vi "sub_font_customize.vi"(0 "REF IN":refnum<vi>, 1 "NOTE":string, 2 "FONT STYLE":T1, 3 "FONT COLOR":cluster{"COLOR":u32, "PHRASE":string[]}[](array[cluster]), 5 "ERROR IN":errorcluster, 8 "HEADER":string, 10 "HEADER EN?":bool) -> (14 "REF OUT":refnum<vi>, 19 "ERROR OUT":errorcluster)   [LabVIEW 2018]
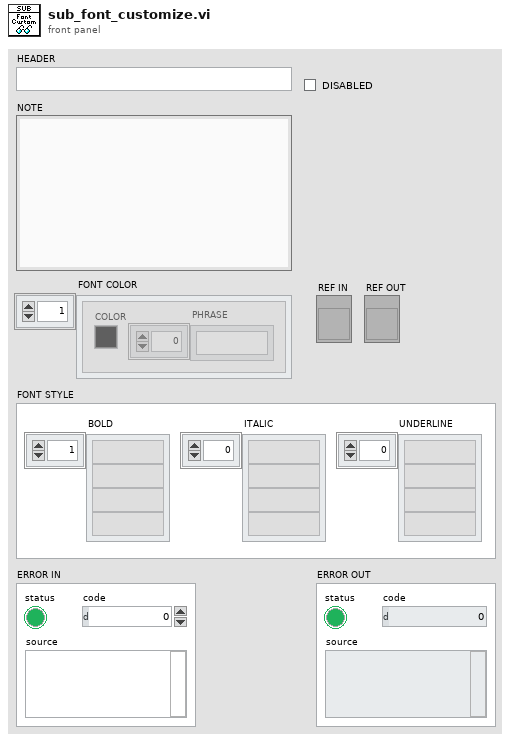
[diagram p1: front panel]
types:
  T1 = cluster{"BOLD":string[], "ITALIC":string[], "UNDERLINE":string[]}
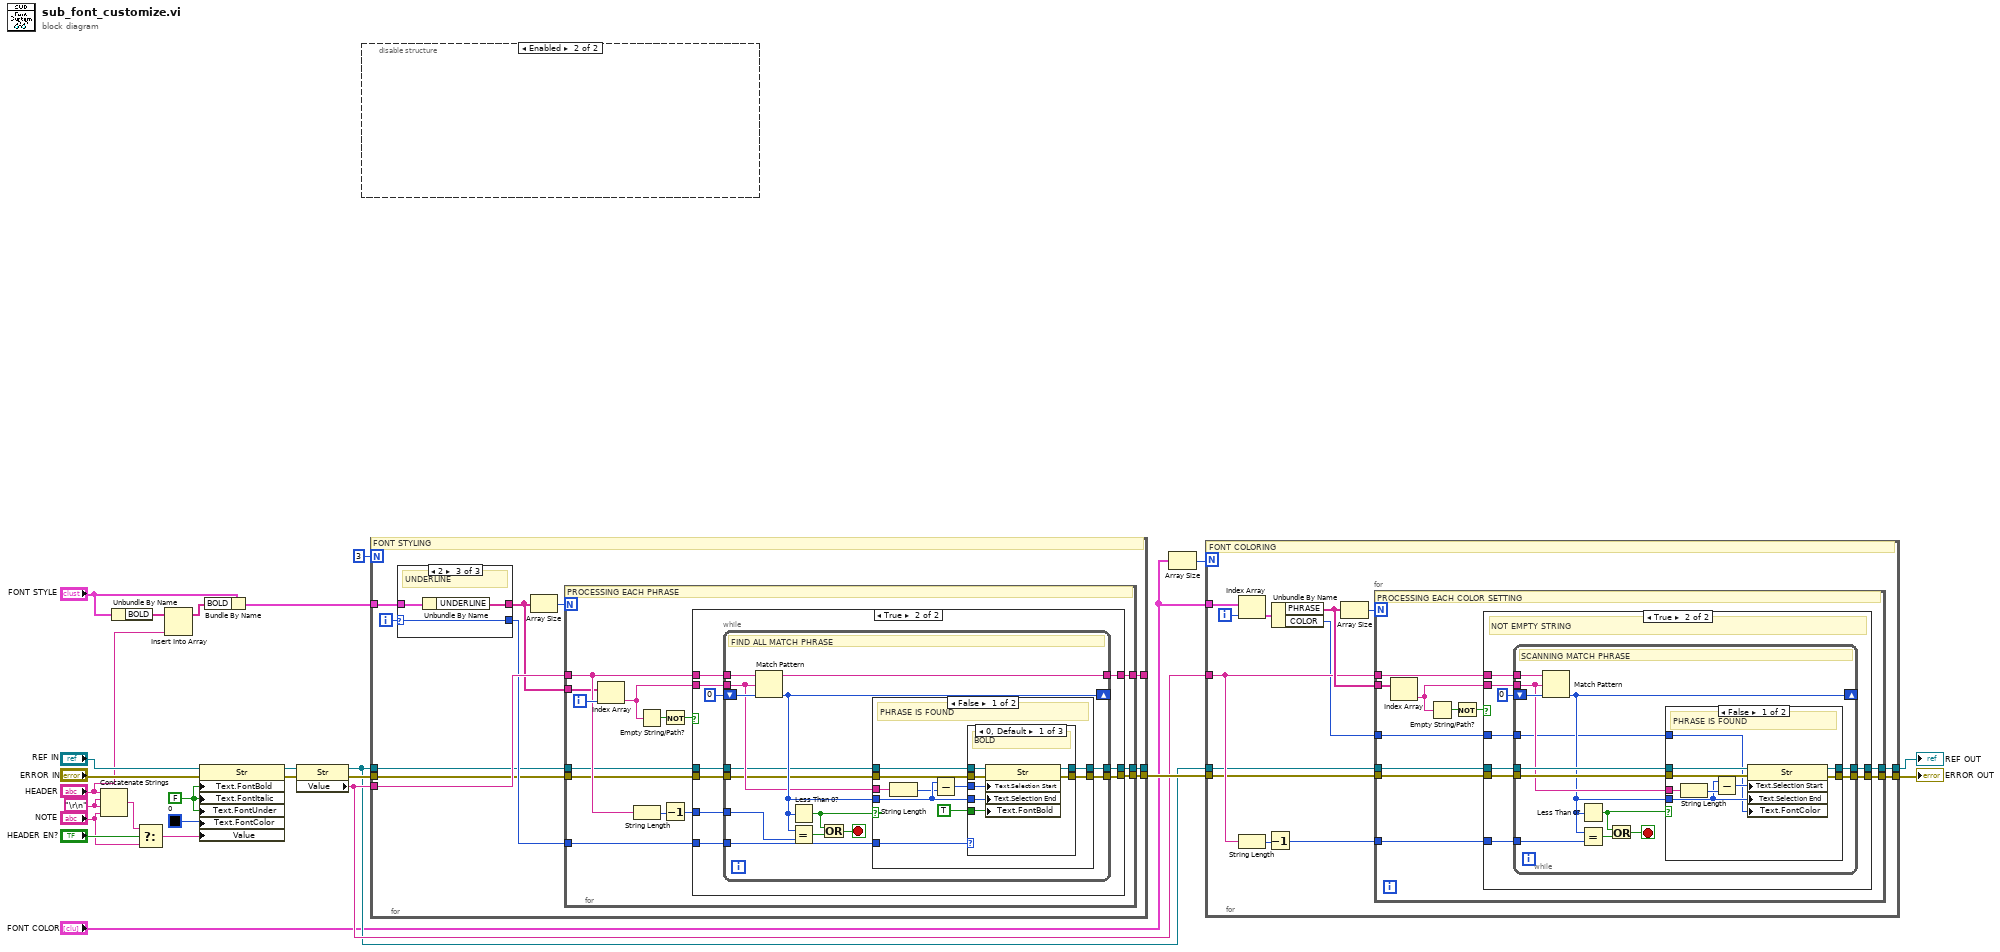
[diagram p0: block diagram]
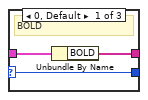
[diagram p4: hidden frame]
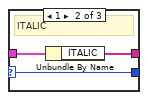
[diagram p5: hidden frame]
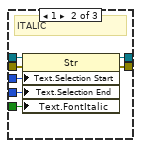
[diagram p7: hidden frame]
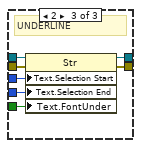
[diagram p8: hidden frame]
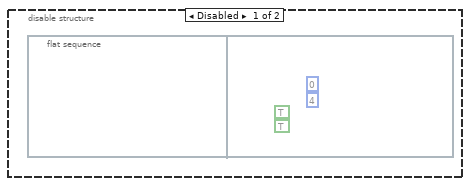
[diagram p10: hidden frame]
diagram:
  w11 = "\r\n"
  w25 = FALSE ("Text.Font:Bold")
  n1 = Concatenate Strings("HEADER", w11, w11, "NOTE") -> (w10:string)
  n2 = Unbundle By Name("FONT STYLE") -> ("BOLD"=w5:string[])
  n3 = Select(t=w10, s="HEADER EN?", f="NOTE") -> (s? t:f=w8:string)
  n4 = Insert Into Array(array=w5, new element="HEADER") -> (w2:string[])  [unwired: 1 in]
  n5 = property on="Property Node" class="Str"(reference="REF IN", error in="ERROR IN", "Text.FontBold"=w25, "Text.FontItalic"=w25, "Text.FontUnder"=w25, "Text.FontColor"=u32 0, "Value"=w8) -> (reference out=w20:refnum<vi>, error out=w23:errorcluster)
  n6 = Bundle By Name(cluster="FONT STYLE", "BOLD"=w2) -> (w1:T1)
  n7 = property on="Property Node" class="Str"(reference=w20, error in=w23) -> (reference out=w15:refnum<vi>, error out=w21:errorcluster, "Value"=w16:string)
  n8 = disable-structure shown="Enabled" {
    frame Disabled {
      n9 = flat-sequence {
        frame #0 {
        }
        frame #1 {
          w26 = TRUE ("Text.Font:Underline")
          w27 = TRUE ("Text.Font:Bold")
          w28 = u32 4 ("Text.Selection:End")
          w29 = u32 0 ("Text.Selection:Start")
        }
      }
    }
    frame Enabled {
    }
  }
  n10 = for {
    N: 3 -> [_]
    tunnel: w16 -> [w40]
    tunnel: w1 -> [w39]
    tunnel: w21 -> [w34]
    tunnel: w15 -> [w33]
    tunnel: [w32] -> _
    tunnel: [w31] -> w18
    tunnel: [w30] -> _
    i -> [w38]
    # "FONT STYLING"
    n11 = case shown="2" w38 {
      selector: w38 -> [w41 w44 w47]
      tunnel: w39 -> [w43 w46 w49]
      tunnel: [w42 w45 w48] -> w36
      tunnel: [w41 w44 w47] -> w37
      frame 0, Default {
        # "BOLD"
        n12 = Unbundle By Name(w43) -> ("BOLD"=w42:string[])
      }
      frame 1 {
        # "ITALIC"
        n13 = Unbundle By Name(w46) -> ("ITALIC"=w45:string[])
      }
      frame 2 {
        # "UNDERLINE"
        n14 = Unbundle By Name(w49) -> ("UNDERLINE"=w48:string[])
      }
    }
    n15 = Array Size(array=w36) -> (size(s)=w35:i32)
    n16 = for {
      N: w35 -> [_]
      tunnel: w40 -> [w60]
      tunnel: w34 -> [w59]
      tunnel: [w58] -> w31
      tunnel: [w57] -> w30
      tunnel: w37 -> [w56]
      tunnel: w36 -> [w55]
      tunnel: w33 -> [w51]
      tunnel: [w50] -> w32
      i -> [w63]
      # "PROCESSING EACH PHRASE"
      n17 = Index Array(array=w55, index=w63) -> (element=w54:string)
      n18 = String Length(string=w60) -> (length=w62:i32)
      n19 = Empty String/Path?(string/path=w54) -> (empty?=w52:bool)
      n20 = Not(x=w52) -> (.not. x?=w53:bool)
      n21 = Decrement(x=w62) -> (x-1=w61:i32)
      n22 = case shown="True" w53 {
        tunnel: w61 -> [_ w76]
        tunnel: w54 -> [_ w75]
        tunnel: w60 -> [w66 w74]
        tunnel: w59 -> [w65 w73]
        tunnel: [w65 w72] -> w58
        tunnel: [w66 w71] -> w57
        tunnel: w56 -> [_ w70]
        tunnel: w51 -> [w64 w69]
        tunnel: [w64 w68] -> w50
        frame False {
        }
        frame True {
          n23 = while {
            tunnel: w74 -> [w80]
            tunnel: w75 -> [w83]
            shift-right: [w84] -> _
            shift-left: 0 ("offset past match") -> [w89]
            tunnel: w76 -> [w88]
            tunnel: [w80] -> w71
            tunnel: w70 -> [w79]
            tunnel: w69 -> [w78]
            tunnel: [w77] -> w68
            tunnel: w73 -> [w81]
            tunnel: [w82] -> w72
            stop <- w86 stop-if-true
            # "FIND ALL MATCH PHRASE"
            n24 = Match Pattern(string=w80, regular expression=w83, offset (0)=w89) -> (offset past match=w84:i32)  [unwired: 3 out]
            n25 = Less Than 0?(x=w84) -> (x < 0?=w85:bool)
            n26 = Equal?(x=w84, y=w88) -> (x = y?=w87:bool)
            n27 = Or(x=w85, y=w87) -> (x .or. y?=w86:bool)
            n28 = case shown="False" w85 {
              tunnel: w84 -> [w97 _]
              tunnel: w83 -> [w96 _]
              tunnel: [w94 w122] -> w82
              tunnel: w81 -> [w93 w122]
              tunnel: w79 -> [w92 _]
              tunnel: w78 -> [w91 w121]
              tunnel: [w90 w121] -> w77
              frame False {
                # "PHRASE IS FOUND"
                n29 = String Length(string=w96) -> (length=w95:i32)
                n30 = Subtract(x=w97, y=w95) -> (x-y=w99:i32)
                n31 = case shown="0, Default" w92 {
                  tunnel: w99 -> [w104 w113 w118]
                  tunnel: TRUE ("Text.Font:Bold") -> [w102 w112 w116]
                  tunnel: w97 -> [w103 w111 w117]
                  tunnel: [w105 w110 w119] -> w94
                  tunnel: w93 -> [w106 w109 w120]
                  tunnel: w91 -> [w101 w108 w115]
                  tunnel: [w100 w107 w114] -> w90
                  frame 0, Default {
                    # "BOLD"
                    n32 = property on="Property Node" class="Str"(reference=w101, error in=w106, "Text.Selection Start"=w104, "Text.Selection End"=w103, "Text.FontBold"=w102) -> (reference out=w100:refnum<vi>, error out=w105:errorcluster)
                  }
                  frame 1 {
                    # "ITALIC"
                    n33 = property on="Property Node" class="Str"(reference=w108, error in=w109, "Text.Selection Start"=w113, "Text.Selection End"=w111, "Text.FontItalic"=w112) -> (reference out=w107:refnum<vi>, error out=w110:errorcluster)
                  }
                  frame 2 {
                    # "UNDERLINE"
                    n34 = property on="Property Node" class="Str"(reference=w115, error in=w120, "Text.Selection Start"=w118, "Text.Selection End"=w117, "Text.FontUnder"=w116) -> (reference out=w114:refnum<vi>, error out=w119:errorcluster)
                  }
                }
              }
              frame True {
                # "PHRASE NOT FOUND"
              }
            }
          }
        }
      }
    }
  }
  n35 = Array Size(array="FONT COLOR") -> (size(s)=w19:i32)
  n36 = for {
    N: w19 -> [_]
    tunnel: w16 -> [w130]
    tunnel: w15 -> [w127]
    tunnel: w18 -> [w126]
    tunnel: "FONT COLOR" -> [w135]
    tunnel: [w124] -> w6
    tunnel: [w123] -> w7
    i -> [w134]
    # "FONT COLORING"
    n37 = Index Array(array=w135, index=w134) -> (element=w133:cluster{"COLOR":u32, "PHRASE":string[]})
    n38 = String Length(string=w130) -> (length=w129:i32)
    n39 = Decrement(x=w129) -> (x-1=w128:i32)
    n40 = Unbundle By Name(w133) -> ("PHRASE"=w131:string[], "COLOR"=w125:u32)
    n41 = Array Size(array=w131) -> (size(s)=w132:i32)
    n42 = for {
      N: w132 -> [_]
      tunnel: w131 -> [w146]
      tunnel: w130 -> [w143]
      tunnel: w128 -> [w141]
      tunnel: w127 -> [w140]
      tunnel: w126 -> [w139]
      tunnel: w125 -> [w138]
      tunnel: [w137] -> w124
      tunnel: [w136] -> w123
      # "PROCESSING EACH COLOR SETTING"
      n43 = Index Array(array=w146) -> (element=w142:string)  [unwired: 1 in]
      n44 = Empty String/Path?(string/path=w142) -> (empty?=w145:bool)
      n45 = Not(x=w145) -> (.not. x?=w144:bool)
      n46 = case shown="True" w144 {
        tunnel: w143 -> [_ w157]
        tunnel: w142 -> [_ w156]
        tunnel: w141 -> [_ w154]
        tunnel: w140 -> [w148 w153]
        tunnel: w139 -> [w147 w152]
        tunnel: w138 -> [_ w151]
        tunnel: [w148 w150] -> w137
        tunnel: [w147 w149] -> w136
        frame False {
          # "EMPTY STRING"
        }
        frame True {
          # "NOT EMPTY STRING"
          n47 = while {
            tunnel: w157 -> [w170]
            tunnel: w156 -> [w162]
            shift-right: [w161] -> _
            shift-left: 0 ("offset past match") -> [w169]
            tunnel: w154 -> [w168]
            tunnel: w153 -> [w164]
            tunnel: w152 -> [w163]
            tunnel: w151 -> [w160]
            tunnel: [w159] -> w150
            tunnel: [w158] -> w149
            stop <- w166 stop-if-true
            # "SCANNING MATCH PHRASE"
            n48 = Match Pattern(string=w170, regular expression=w162, offset (0)=w169) -> (offset past match=w161:i32)  [unwired: 3 out]
            n49 = Less Than 0?(x=w161) -> (x < 0?=w165:bool)
            n50 = Equal?(x=w161, y=w168) -> (x = y?=w167:bool)
            n51 = Or(x=w165, y=w167) -> (x .or. y?=w166:bool)
            n52 = case shown="False" w165 {
              tunnel: w164 -> [w179 w181]
              tunnel: w163 -> [w178 w180]
              tunnel: w162 -> [w177 _]
              tunnel: w161 -> [w174 _]
              tunnel: w160 -> [w173 _]
              tunnel: [w172 w181] -> w159
              tunnel: [w171 w180] -> w158
              frame False {
                # "PHRASE IS FOUND"
                n53 = String Length(string=w177) -> (length=w176:i32)
                n54 = Subtract(x=w174, y=w176) -> (x-y=w175:i32)
                n55 = property class="Str"(reference=w179, error in=w178, "Text.Selection Start"=w175, "Text.Selection End"=w174, "Text.FontColor"=w173) -> (reference out=w172:refnum<vi>, error out=w171:errorcluster)
              }
              frame True {
                # "PHRASE NOT FOUND"
              }
            }
          }
        }
      }
    }
  }
  "REF OUT" <- w6
  "ERROR OUT" <- w7
